vi "sliderClose.vi"() -> (0 "error out":errorcluster)   [LabVIEW 2017]
uses:
  globalDevices.vi
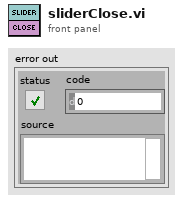
[diagram p1: front panel]
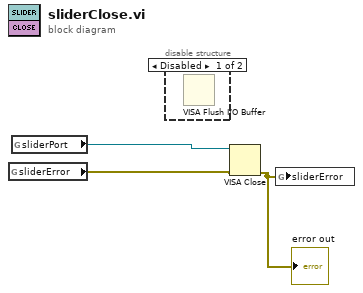
[diagram p0: block diagram]
diagram:
  n1 = global read "globalDevices.vi" "sliderError"() -> (w1:errorcluster)
  n2 = global read "globalDevices.vi" "sliderPort"() -> (w2:refnum<visa-resource-name>)
  n3 = disable-structure shown="Disabled" {
    frame Disabled {
      n4 = VISA Flush I/O Buffer() -> ()  [unwired: 3 in, 2 out]
    }
    frame Enabled {
    }
  }
  n5 = VISA Close(VISA resource name=w2, error in (no error)=w1) -> (error out=w3:errorcluster)
  "error out" <- w3
  n6 = global write "globalDevices.vi" "sliderError"(w3) -> ()
